vi "new.vi"() -> ()   [LabVIEW 2020]
panel:
  in  "Numeric 1":dbl
  in  "Boolean":bool
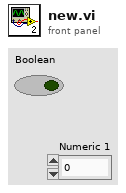
[diagram p1: front panel]
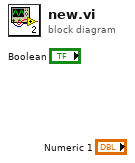
[diagram p0: block diagram]
diagram:
